vi "Multiple Calls.vi"(8 "For loop index":i32, 9 "Maximum Items per Request":u16, 10 "Item offset [byte]":u32, 11 "items #":u16) -> (0 "Items left (shift register)":u16, 1 "Result Array offset":i32, 2 "Item Offset":u32, 3 "Items to read":u16)   [LabVIEW 2014, in "Simatic S7.lvlib"]
uses:
  Simatic S7.lvlib
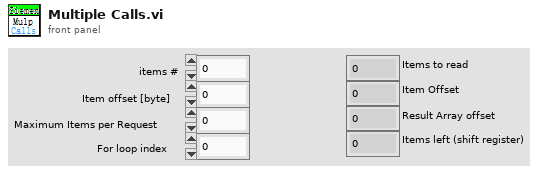
[diagram p1: front panel]
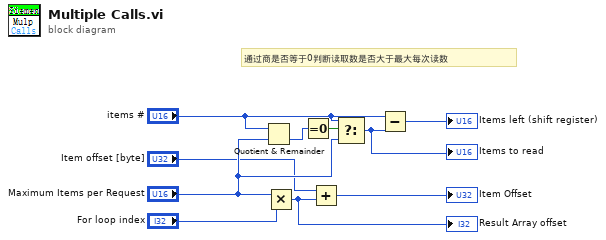
[diagram p0: block diagram]
diagram:
  # "通过商是否等于0判断读取数是否大于最大每次读数"
  n1 = Quotient & Remainder(x="items #", y="Maximum Items per Request") -> (floor(x/y)=w7:u16)  [unwired: 1 out]
  n2 = Multiply(x="Maximum Items per Request", y="For loop index") -> (x*y=w8:i32)
  "Result Array offset" <- w8
  n3 = Equal To 0?(x=w7) -> (x = 0?=w3:bool)
  n4 = Add(x="Item offset [byte]", y=w8) -> (x+y=→"Item Offset":u32)
  n5 = Select(t="items #", s=w3, f="Maximum Items per Request") -> (s? t:f=w5:u16)
  "Items to read" <- w5
  n6 = Subtract(x="items #", y=w5) -> (x-y=→"Items left (shift register)":u16)
